vi "KE26XX Config Source & Measure.vi"(3 "Error Query (False)":bool, 4 "Limit":dbl=1.0, 5 "Measure Function (Current)":T2(ring), 6 "Level":dbl=1.0, 7 "Source Function (Current)":enum32{"Current", "Voltage"}(ring)=enum."Voltage", 8 "error in (no error)":errorcluster, 9 "Channel (Channel A)":T1, 10 "Node (0-64)":i8 min=0 max=64 step=1, 11 "VISA resource name":refnum<visa-resource-name>) -> (0 "error out":errorcluster, 1 "Output":string)   [LabVIEW 2012]
doc: "This example shows how to configure the source and take a measurement."
uses:
  Keithley 2600 Series.lvlib
  Public/Channel.ctl
panel:
  in  "stop":bool
  in  "Channel (Channel A) 2":T1
  in  "Source Function (Current) 2":enum32{"Current", "Voltage"}(ring)=enum."Voltage"
  in  "Limit 2":dbl=1.0
  in  "Level 2":dbl=1.0
  in  "Measure Function (Current) 2":T2(ring)
  out "Output 2":string
  # "(c) 2008 Keithley Instruments, Inc.  ALL RIGHTS RESERVED."
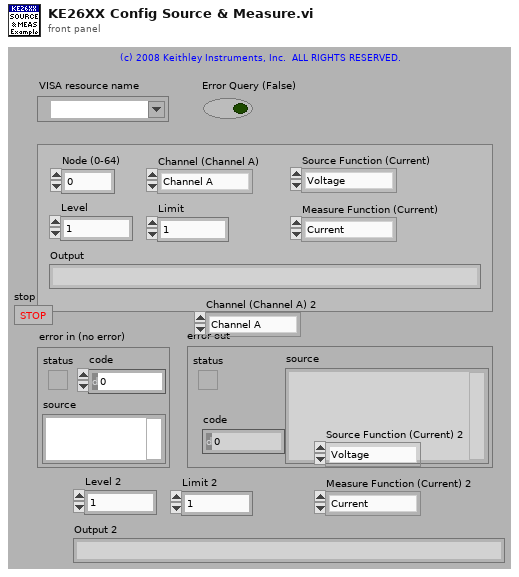
[diagram p1: front panel]
types:
  T1 = typedef "Keithley 2600 Series.lvlib/Channel.ctl" = enum32{"Channel A", "Channel B"}
  T2 = enum32{"Current", "Voltage", "IV", "Resistance", "Power"}
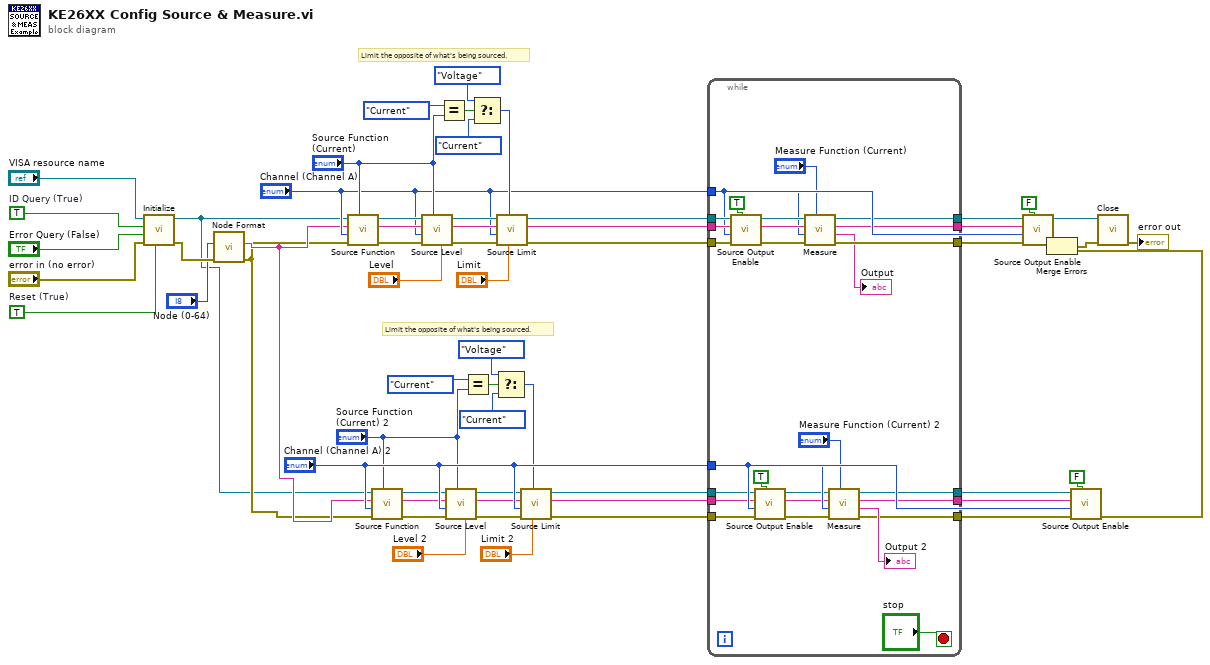
[diagram p0: block diagram]
diagram:
  w40 = TRUE  # Reset (True)
  w57 = TRUE  # ID Query (True)
  # "Limit the opposite of what's being sourced."
  # "Limit the opposite of what's being sourced."
  n1 = call "Initialize.vi"("Reset (True)"=w40, "error in (no error)"="error in (no error)", "Error Query (False)"="Error Query (False)", "ID Query (True)"=w57, "VISA resource name"="VISA resource name") -> ("error out"=w32:errorcluster, "VISA resource name out"=w4:refnum<visa-resource-name>)  [unwired: 1 in, 4 out]
  n2 = call "Node Format.vi"("error in"=w32, "Node (0-64)"="Node (0-64)") -> ("error out"=w5:errorcluster, "Formatted Node"=w6:string)  [unwired: 8 out]
  n3 = call "Source Function.vi"("Function (Current)"="Source Function (Current)", "error in (no error)"=w5, "Channel (Channel A)"="Channel (Channel A)", "Node In"=w6, "VISA resource name"=w4) -> ("error out"=w53:errorcluster, "Node Out"=w55:string, "VISA resource name out"=w54:refnum<visa-resource-name>)  [unwired: 4 out]
  n4 = call "Source Function.vi"("Function (Current)"="Source Function (Current) 2", "error in (no error)"=w5, "Channel (Channel A)"="Channel (Channel A) 2", "Node In"=w6, "VISA resource name"=w4) -> ("error out"=w9:errorcluster, "Node Out"=w7:string, "VISA resource name out"=w8:refnum<visa-resource-name>)  [unwired: 4 out]
  n5 = call "Source Level.vi"("Level (0.000)"="Level", "Function (Current)"="Source Function (Current)", "error in (no error)"=w53, "Channel (Channel A)"="Channel (Channel A)", "Node In"=w55, "VISA resource name"=w54) -> ("error out"=w52:errorcluster, "Node Out"=w43:string, "VISA resource name out"=w51:refnum<visa-resource-name>)  [unwired: 3 out]
  n6 = Equal?(x=enum32{"Current", "Voltage"}."Current", y="Source Function (Current)") -> (x = y?=w37:bool)
  n7 = call "Source Level.vi"("Level (0.000)"="Level 2", "Function (Current)"="Source Function (Current) 2", "error in (no error)"=w9, "Channel (Channel A)"="Channel (Channel A) 2", "Node In"=w7, "VISA resource name"=w8) -> ("error out"=w10:errorcluster, "Node Out"=w17:string, "VISA resource name out"=w11:refnum<visa-resource-name>)  [unwired: 3 out]
  n8 = Equal?(x=enum32{"Current", "Voltage"}."Current", y="Source Function (Current) 2") -> (x = y?=w22:bool)
  n9 = Select(t=enum32{"Current", "Voltage"}."Voltage" ("x"), s=w37, f=enum32{"Current", "Voltage"}."Current") -> (s? t:f=w35:enum32{"Current", "Voltage"})
  n10 = Select(t=enum32{"Current", "Voltage"}."Voltage" ("x"), s=w22, f=enum32{"Current", "Voltage"}."Current") -> (s? t:f=w24:enum32{"Current", "Voltage"})
  n11 = call "Source Limit.vi"("Limit (0.000)"="Limit", "Function (Current)"=w35, "error in (no error)"=w52, "Channel (Channel A)"="Channel (Channel A)", "Node In"=w43, "VISA resource name"=w51) -> ("error out"=w49:errorcluster, "Node Out"=w42:string, "VISA resource name out"=w50:refnum<visa-resource-name>)  [unwired: 3 out]
  n12 = call "Source Limit.vi"("Limit (0.000)"="Limit 2", "Function (Current)"=w24, "error in (no error)"=w10, "Channel (Channel A)"="Channel (Channel A) 2", "Node In"=w17, "VISA resource name"=w11) -> ("error out"=w13:errorcluster, "Node Out"=w18:string, "VISA resource name out"=w12:refnum<visa-resource-name>)  [unwired: 3 out]
  n13 = while {
    tunnel: w50 -> [w86]
    tunnel: w49 -> [w85]
    tunnel: [w82] -> w48
    tunnel: [w81] -> w47
    tunnel: w42 -> [w79]
    tunnel: [w77] -> w41
    tunnel: "Channel (Channel A)" -> [w74]
    tunnel: "Channel (Channel A) 2" -> [w73]
    tunnel: [w70] -> w19
    tunnel: w18 -> [w68]
    tunnel: [w66] -> w15
    tunnel: [w65] -> w14
    tunnel: w13 -> [w62]
    tunnel: w12 -> [w61]
    stop <- "stop" stop-if-true
    n14 = call "Source Output Enable.vi"("Output (Off)"=TRUE, "error in (no error)"=w85, "Channel (Channel A)"=w74, "Node In"=w79, "VISA resource name"=w86) -> ("error out"=w84:errorcluster, "Node Out"=w78:string, "VISA resource name out"=w83:refnum<visa-resource-name>)  [unwired: 4 out]
    n15 = call "Source Output Enable.vi"("Output (Off)"=TRUE, "error in (no error)"=w62, "Channel (Channel A)"=w73, "Node In"=w68, "VISA resource name"=w61) -> ("error out"=w63:errorcluster, "Node Out"=w69:string, "VISA resource name out"=w64:refnum<visa-resource-name>)  [unwired: 4 out]
    n16 = call "Measure.vi"("Function (Current)"="Measure Function (Current)", "error in (no error)"=w84, "Channel (Channel A)"=w74, "Node In"=w78, "VISA resource name"=w83) -> ("error out"=w81:errorcluster, "Output"=→"Output":string, "Node Out"=w77:string, "VISA resource name out"=w82:refnum<visa-resource-name>)  [unwired: 2 in, 1 out]
    n17 = call "Measure.vi"("Function (Current)"="Measure Function (Current) 2", "error in (no error)"=w63, "Channel (Channel A)"=w73, "Node In"=w69, "VISA resource name"=w64) -> ("error out"=w66:errorcluster, "Output"=→"Output 2":string, "Node Out"=w70:string, "VISA resource name out"=w65:refnum<visa-resource-name>)  [unwired: 2 in, 1 out]
  }
  n18 = call "Source Output Enable.vi"("Output (Off)"=FALSE, "error in (no error)"=w47, "Channel (Channel A)"="Channel (Channel A)", "Node In"=w41, "VISA resource name"=w48) -> ("error out"=w2:errorcluster, "VISA resource name out"=w46:refnum<visa-resource-name>)  [unwired: 5 out]
  n19 = call "Source Output Enable.vi"("Output (Off)"=FALSE, "error in (no error)"=w15, "Channel (Channel A)"="Channel (Channel A) 2", "Node In"=w19, "VISA resource name"=w14) -> ("error out"=w1:errorcluster)  [unwired: 6 out]
  n20 = Merge Errors(w2, w1) -> (w3:errorcluster)
  n21 = call "Close.vi"("error in (no error)"=w3, "VISA resource name"=w46) -> ("error out"=→"error out":errorcluster)  [unwired: 9 out]
